vi "Get DH Convention.vi"(8 "error in (no error)":errorcluster, 11 "Link In":refnum<class "NI_Robotics_Link.lvclass">) -> (0 "error out":errorcluster, 2 "DH Convention":T1, 3 "Link Out":refnum<class "NI_Robotics_Link.lvclass">)   [LabVIEW 2017, in "NI_Robotics_Link.lvclass"]
uses:
  <vilib>/robotics/Kinematics/Link/NI_Robotics_Link.lvclass
  <vilib>/robotics/Kinematics/DH Convention.ctl
  <vilib>/robotics/Kinematics/Link/NI_Robotics_Link.lvclass/NI_Robotics_Link.ctl
  <vilib>/robotics/Kinematics/NI_Kinematics.lvlib
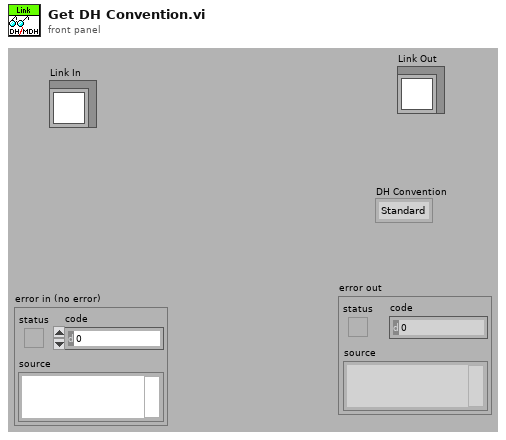
[diagram p1: front panel]
types:
  T1 = typedef "NI_Kinematics.lvlib/DH Convention.ctl" = enum16{"Standard", "Modified"}
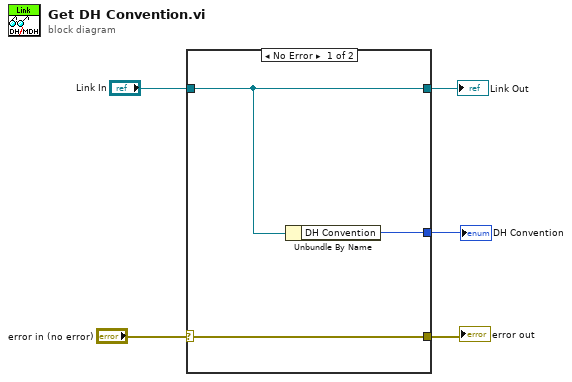
[diagram p0: block diagram]
diagram:
  n1 = case shown="No Error" "error in (no error)" {
    selector: "error in (no error)" -> [w6 w9]
    tunnel: "Link In" -> [w7 w10]
    tunnel: [w8 _] -> w4
    tunnel: [w7 w10] -> w3
    tunnel: [w6 w9] -> w1
    frame No Error {
      n2 = Unbundle By Name(w7) -> ("DH Convention"=w8:T1)
    }
    frame Error {
    }
  }
  "Link Out" <- w3
  "DH Convention" <- w4
  "error out" <- w1
